vi "GetContextHelpInfo.vi"(0 "reference in":refnum<class "VINode.lvclass">, 1 "MousePos":T1 {"y" format="%.2f"; "x" format="%.2f"}, 5 "error in (no error)":errorcluster) -> (14 "reference out":refnum<class "VINode.lvclass">, 15 "ContextHelpInfoExist":bool, 16 "ContextHelpInfo":variant, 19 "error out":errorcluster)   [LabVIEW 2014, in "VINode.lvclass"]
doc: "GetContextHelpInfo"
uses:
  <resource>/Framework/Providers/Open_GDS/UML/VINode_class/VINode.lvclass
  <resource>/Framework/Providers/Open_GDS/UML/General/Point/Point Point2D.ctl
  <resource>/Framework/Providers/Open_GDS/UML/MultiLineString_class/MultiLineString.lvclass
  <resource>/Framework/Providers/Open_GDS/UML/RectangularNode_class/RectangularNode.lvclass
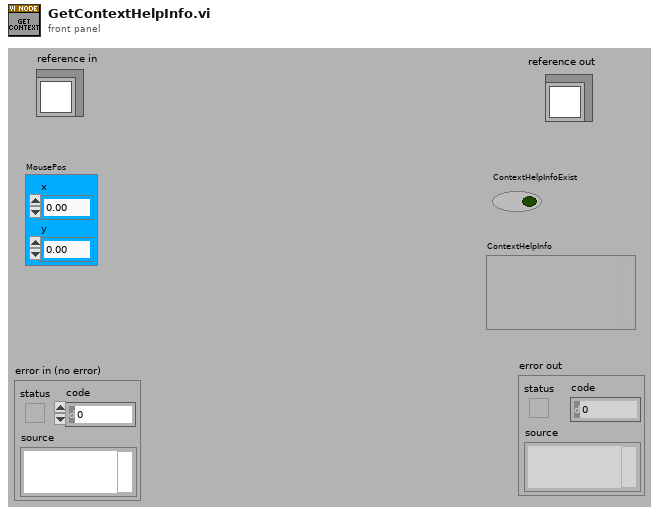
[diagram p1: front panel]
types:
  T1 = typedef "Point Point2D.ctl" = cluster{"x":dbl, "y":dbl}
  T2 = typedef "VINode.lvclass/ObjectAttributes.ctl" = cluster{"midHeight":dbl, "botHeight":dbl, "Name":refnum<class "MultiLineString.lvclass">, "DEFAULT_COMPARTMENT_HEIGHT":i32, "DEFAULT_WIDTH":i32, "DEFAULT_HEIGHT":i32, "ClassPath":path, "Icon":u8[][], "Description":refnum<class "MultiLineString.lvclass">, "ShowDescription":bool}
  T3 = typedef "RectangularNode.lvclass/ObjectAttributes.ctl" = cluster{"bounds":T4}
  T4 = typedef "Rectangle Rectangle2D.ctl" = cluster{"x":dbl, "y":dbl, "width":dbl, "height":dbl}
  T5 = cluster{"text":string, "empty picture":picture, "Description":string}
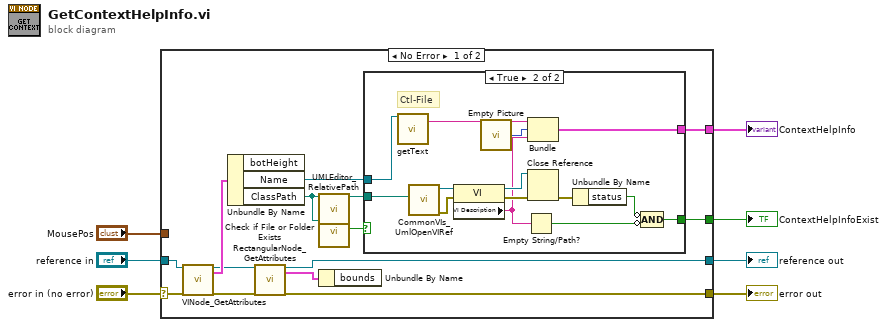
[diagram p0: block diagram]
diagram:
  n1 = case shown="No Error" "error in (no error)" {
    selector: "error in (no error)" -> [w21 w36]
    tunnel: "reference in" -> [w20 w37]
    tunnel: [w8 w36] -> w5
    tunnel: [w12 w37] -> w4
    tunnel: "MousePos" -> [_ _]
    tunnel: [w19 _] -> w2
    tunnel: [w18 _] -> w1
    frame No Error {
      n2 = call <resource>:"VINode_GetAttributes.vi"("reference in"=w20, "error in (no error)"=w21) -> ("reference out"=w14:refnum<class "VINode.lvclass">, "Data"=w15:T2, "error out"=w13:errorcluster)  [unwired: 1 in, 14 out]
      n3 = Unbundle By Name(w15) -> ("Name"=w17:refnum<class "MultiLineString.lvclass">, "ClassPath"=w10:path)  [unwired: 1 out]
      n4 = call <resource>:"RectangularNode_GetAttributes.vi"("reference in"=w14, "error in (no error)"=w13) -> ("reference out"=w12:refnum<class "VINode.lvclass">, "Data"=w11:T3, "error out"=w8:errorcluster)  [unwired: 14 in, 1 out]
      n5 = call <resource>:"UMLEditor_RelativePath.vi"("Path In"=w10) -> ("ConvertToAbsolutePath(If possible)"=w16:path)  [unwired: 1 in, 17 out]
      n6 = call <vilib>:"Check if File or Folder Exists.vi"("path"=w10) -> ("file or folder exists?"=w9:bool)  [unwired: 8 in, 2 out]
      n7 = Unbundle By Name(w11) -> ()  [unwired: 1 out]
      n8 = case shown="True" w9 {
        tunnel: [_ w28] -> w19
        tunnel: [_ w30] -> w18
        tunnel: w16 -> [_ w23]
        tunnel: w17 -> [_ w27]
        frame False {
        }
        frame True {
          # "Ctl-File"
          n9 = call-dynamic "getText.vi"("reference"=w27) -> ("text"=w26:string)  [unwired: 1 in, 17 out]
          n10 = call <resource>:"CommonVIs_UmlOpenVIRef.vi"("ViPath/ViName"=w23) -> ("error out"=w22:errorcluster, "vi reference"=w24:refnum<vi>)  [unwired: 7 in, 2 out]
          n11 = property class="VI"(reference=w24, error in=w22) -> (reference out=w35:refnum<vi>, error out=w34:errorcluster, "VI Description"=w25:string)
          n12 = call "Empty Picture"() -> ("empty picture"=w29:picture)
          n13 = Empty String/Path?(string/path=w25) -> (empty?=w31:bool)
          n14 = Bundle("text"=w26, "empty picture"=w29, "Description"=w25) -> (w28:T5)  [unwired: 1 out]
          n15 = Close Reference(reference=w35, error in (no error)=w34) -> (error out=w33:errorcluster)
          n16 = Unbundle By Name(w33) -> ("status"=w32:bool)
          n17 = Compound Arithmetic op=AND(invert w32, invert w31) -> (w30:bool)
        }
      }
    }
    frame Error {
    }
  }
  "reference out" <- w4
  "error out" <- w5
  "ContextHelpInfo" <- w2
  "ContextHelpInfoExist" <- w1
